vi "Configure Active Trace.vi"(5 "Format":T1, 7 "S parameter":T2(ring), 8 "error in (no error)":errorcluster, 10 "Active Trace":u8=1, 11 "Vector Network Analyzer in":refnum<class "Vector Network Analyzer.lvclass">) -> (0 "error out":errorcluster, 3 "Vector Network Analyzer out":refnum<class "Vector Network Analyzer.lvclass">)   [LabVIEW 2020, in "Vector Network Analyzer.lvclass"]
doc: "Configures the active trace.\nIt creates the trace and sets the S paramert and mode."
uses:
  Vector Network Analyzer.lvclass
  Controls/S parm format enum.ctl
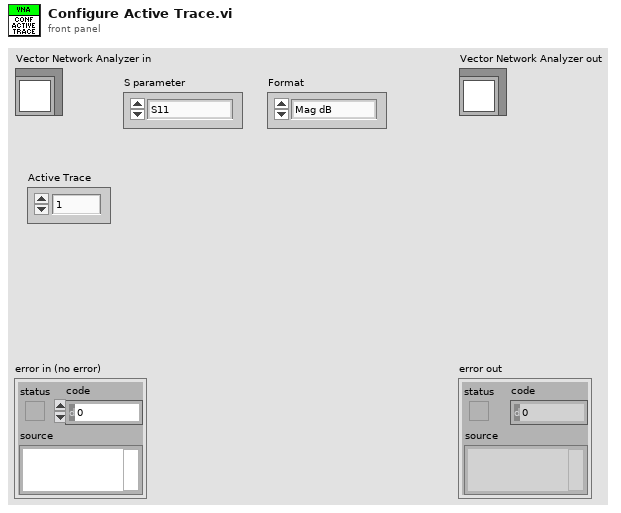
[diagram p1: front panel]
types:
  T1 = typedef "Vector Network Analyzer.lvclass/S parm format enum.ctl" = enum16{"Mag dB", "Mag", "Phase", "Smith", "Real", "Imag", "Group Delay", "SWR"}
  T2 = enum16{"S11", "S21", "S31", "S41", "S22", "S12", "S32", "S42", "S33", "S13", "S23", "S43", "S44", "S14", "S24", "S34"}
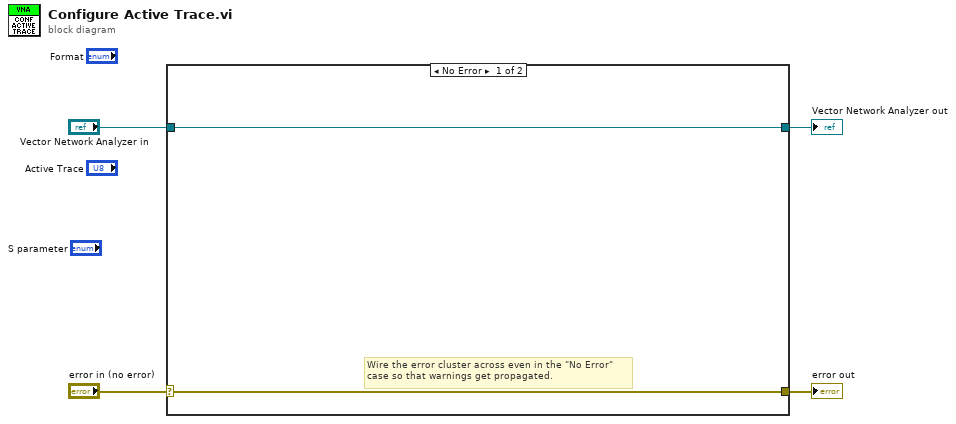
[diagram p0: block diagram]
diagram:
  n1 = case shown="No Error" "error in (no error)" {
    selector: "error in (no error)" -> [w5 w8]
    tunnel: [w5 w8] -> w3
    tunnel: [w6 w7] -> w1
    tunnel: "Vector Network Analyzer in" -> [w6 w7]
    frame No Error {
      # "Wire the error cluster across even in the \"No Error\"\ncase so that warnings get propagated."
    }
    frame Error {
    }
  }
  "error out" <- w3
  "Vector Network Analyzer out" <- w1
